vi "Power-config.vi"(8 "error in (no error)":errorcluster, 11 "powermeter in":refnum<vi>) -> (0 "error out":errorcluster)   [LabVIEW 2016]
uses:
  controls/powermeter.ctl
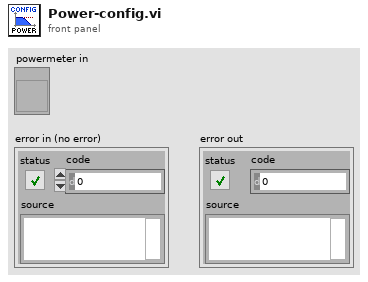
[diagram p1: front panel]
types:
  T1 = typedef "powermeter.ctl" = cluster{"Start":bool, "Serial ":string, "Model":string, "Sensor":string, "Power":dbl, "Density":bool, "Lambda":dbl, "Open":bool, "Save":bool, "reference":refnum<k7>, "hDevice":i32, "Dev. Std.":dbl, "Channel":i16}
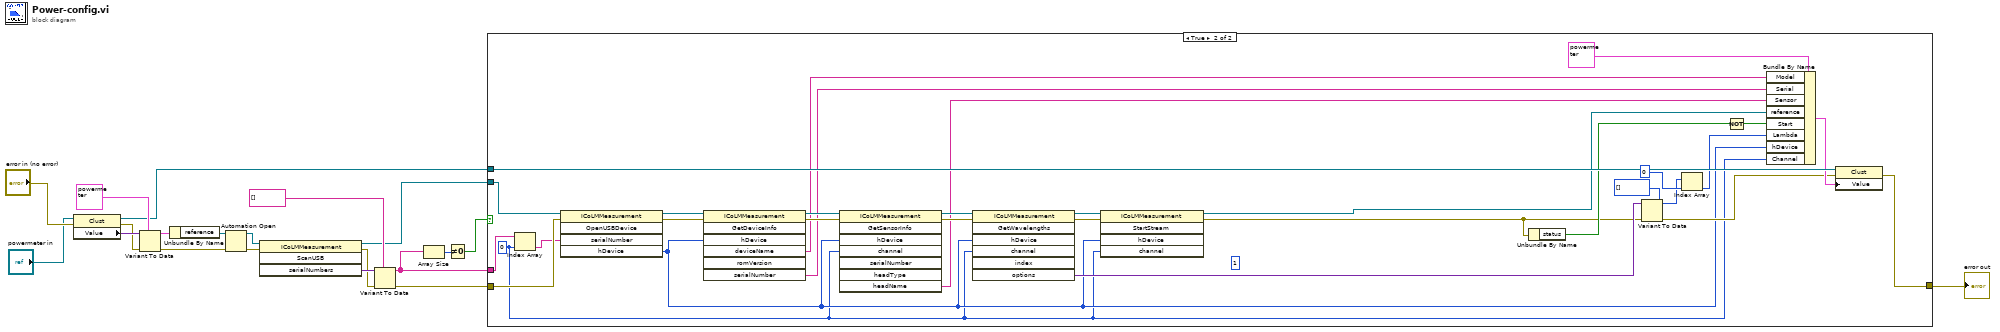
[diagram p0: block diagram]
diagram:
  n1 = property class="Clust"(reference="powermeter in", error in="error in (no error)") -> (reference out=w3:refnum<vi>, error out=w10:errorcluster, "Value"=w11:variant)
  n2 = Variant To Data(error in=w10, type=T1 {"Start"=FALSE, "Serial "="", "Model"="", "Sensor"="", "Power"=0.0, "Density"=FALSE, "Lambda"=0.0, "Open"=FALSE, "Save"=FALSE, "reference"=refnum, "hDevice"=0, "Dev. Std."=0.0, "Channel"=0} ("Power Meter"), Variant=w11) -> (data=w13:T1, error out=w15:errorcluster)
  n3 = Unbundle By Name(w13) -> ("reference"=w14:refnum<k7>)
  n4 = Automation Open(error in (no error)=w15, Automation Refnum=w14) -> (Automation Refnum=w17:refnum<k7>, error out=w16:errorcluster)  [unwired: 2 in]
  n5 = invoke class="ICoLMMeasurement" method="ScanUSB"(reference=w17, error in=w16) -> (reference out=w2:refnum<k7>, error out=w18:errorcluster, "serialNumbers"=w19:variant)  [unwired: 2 in, 1 out]
  n6 = Variant To Data(error in=w18, type=string[] [], Variant=w19) -> (data=w1:string[], error out=w5:errorcluster)
  n7 = Array Size(array=w1) -> (size(s)=w7:i32)
  n8 = Not Equal To 0?(x=w7) -> (x != 0?=w6:bool)
  n9 = case shown="True" w6 {
    tunnel: w5 -> [w21 w50]
    tunnel: w1 -> [_ w52]
    tunnel: w2 -> [_ w51]
    tunnel: [w21 w30] -> w4
    tunnel: w3 -> [_ w38]
    frame False {
    }
    frame True {
      (unwired) 1 ("index")
      w24 = 0
      n10 = Index Array(array=w52, index=w24) -> (element=w49:string)
      n11 = invoke class="ICoLMMeasurement" method="OpenUSBDevice"(reference=w51, error in=w50, "serialNumber"=w49) -> (reference out=w48:refnum<k7>, error out=w47:errorcluster, "hDevice"=w25:i32)  [unwired: 2 in, 2 out]
      n12 = invoke class="ICoLMMeasurement" method="GetDeviceInfo"(reference=w48, error in=w47, "hDevice"=w25) -> (reference out=w46:refnum<k7>, error out=w45:errorcluster, "deviceName"=w36:string, "serialNumber"=w35:string)  [unwired: 4 in, 3 out]
      n13 = invoke class="ICoLMMeasurement" method="GetSensorInfo"(reference=w46, error in=w45, "hDevice"=w25, "channel"=w24) -> (reference out=w44:refnum<k7>, error out=w43:errorcluster, "headName"=w33:string)  [unwired: 4 in, 5 out]
      n14 = invoke class="ICoLMMeasurement" method="GetWavelengths"(reference=w44, error in=w43, "hDevice"=w25, "channel"=w24) -> (reference out=w29:refnum<k7>, error out=w28:errorcluster, "options"=w39:variant)  [unwired: 3 in, 4 out]
      n15 = invoke class="ICoLMMeasurement" method="StartStream"(reference=w29, error in=w28, "hDevice"=w25, "channel"=w24) -> (reference out=w23:refnum<k7>, error out=w22:errorcluster)  [unwired: 1 in, 3 out]
      n16 = Unbundle By Name(w22) -> ("status"=w26:bool)
      n17 = Variant To Data(error in=w22, type=i32[] [], Variant=w39) -> (data=w41:i32[], error out=w31:errorcluster)
      n18 = Index Array(array=w41, index=0) -> (element=w32:i32)
      n19 = Not(x=w26) -> (.not. x?=w27:bool)
      n20 = Bundle By Name(cluster=T1 {"Start"=FALSE, "Serial "="", "Model"="", "Sensor"="", "Power"=0.0, "Density"=FALSE, "Lambda"=0.0, "Open"=FALSE, "Save"=FALSE, "reference"=refnum, "hDevice"=0, "Dev. Std."=0.0, "Channel"=0} ("POWER METER in"), "Model"=w36, "Serial"=w35, "Sensor"=w33, "reference"=w23, "Start"=w27, "Lambda"=w32, "hDevice"=w25, "Channel"=w24) -> (w34:T1)
      n21 = property class="Clust"(reference=w38, error in=w31, "Value"=w34) -> (error out=w30:errorcluster)  [unwired: 1 out]
    }
  }
  "error out" <- w4
